vi "Set Voltage and Current.vi"(0 "Tektronix PA1000 in":refnum<class "Tektronix PA1000.lvclass">, 5 "Card #":u8, 7 "Voltage enum number":u16, 9 "Current enum number":u16, 11 "error in (no error)":errorcluster) -> (4 "Tektronix PA1000 out":refnum<class "Tektronix PA1000.lvclass">, 15 "error out":errorcluster)   [LabVIEW 2013, in "Universal Power Meter.lvlib" / "Tektronix PA1000.lvlib" / "Tektronix PA1000.lvclass"]
uses:
  Tektronix PA1000.lvclass
  Universal Power Meter class/Universal Power Meter.lvclass
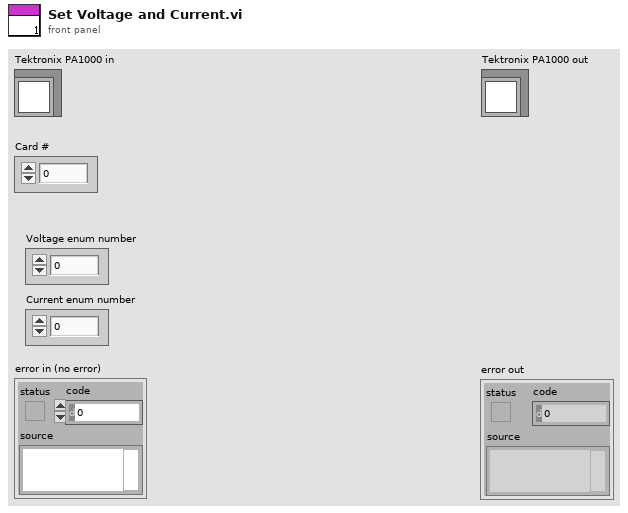
[diagram p1: front panel]
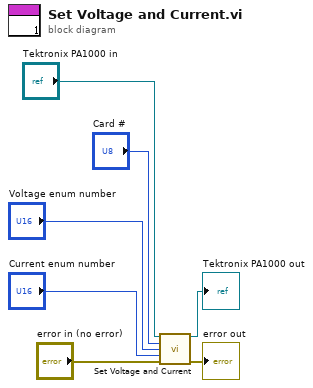
[diagram p0: block diagram]
diagram:
  n1 = call-parent "Set Voltage and Current.vi"("Universal Power Meter in"="Tektronix PA1000 in", "Card #"="Card #", "Voltage enum number"="Voltage enum number", "Current enum number"="Current enum number", "error in (no error)"="error in (no error)") -> ("Universal Power Meter out"=→"Tektronix PA1000 out":refnum<class "Tektronix PA1000.lvclass">, "error out"=→"error out":errorcluster)  [unwired: 9 in]
